vi "Create File and Subfolders.vi"(8 "error in (no error)":errorcluster, 11 "filepath":path) -> (0 "error out":errorcluster)   [LabVIEW 2014]
doc: "Create file and subfolders if they do not already exist."
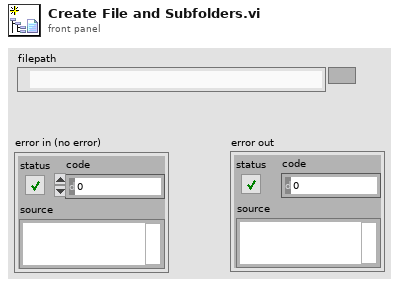
[diagram p1: front panel]
types:
  T1 = enum16{"open", "replace", "create", "open or create", "replace or create", "replace or create with confirmation"}
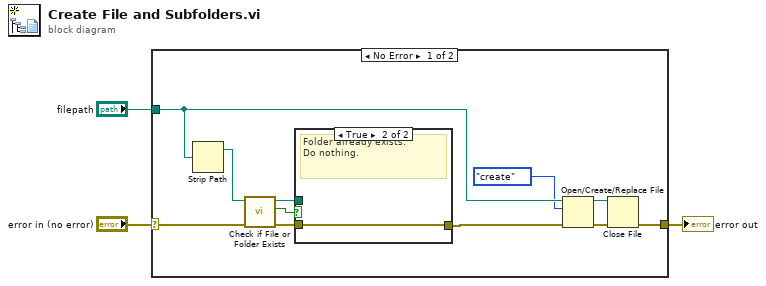
[diagram p0: block diagram]
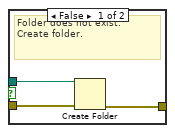
[diagram p2: hidden frame]
diagram:
  n1 = case shown="No Error" "error in (no error)" {
    selector: "error in (no error)" -> [w4 w19]
    tunnel: [w14 w19] -> w3
    tunnel: "filepath" -> [w13 _]
    frame No Error {
      n2 = Strip Path(path=w13) -> (stripped path=w9:path)  [unwired: 1 out]
      n3 = call <vilib>:"Check if File or Folder Exists.vi"("error in (no error)"=w4, "path"=w9) -> ("error out"=w7:errorcluster, "file or folder exists?"=w8:bool, "dup path"=w6:path)  [unwired: 7 in]
      n4 = case shown="True" w8 {
        tunnel: w7 -> [w17 w18]
        tunnel: w6 -> [w16 _]
        tunnel: [w15 w18] -> w5
        frame False {
          # "Folder does not exist.  Create folder."
          n5 = Create Folder(path (use dialog)=w16, error in=w17) -> (error out=w15:errorcluster)  [unwired: 1 in, 2 out]
        }
        frame True {
          # "Folder already exists.\nDo nothing."
        }
      }
      n6 = Open/Create/Replace File(file path (use dialog)=w13, error in=w5, operation (0:open)=T1."create") -> (refnum out=w10:refnum<file>, error out=w11:errorcluster)  [unwired: 3 in, 1 out]
      n7 = Close File(refnum=w10, error in=w11) -> (error out=w14:errorcluster)  [unwired: 1 out]
    }
    frame Error {
    }
  }
  "error out" <- w3
